vi "QuitTest.vi"(8 "error in":errorcluster caption="错误输入（无错误）", 11 "Com":refnum<visa-resource-name>) -> (0 "error out":errorcluster caption="错误输出", 3 "OK?":bool)   [LabVIEW 2013]
uses:
  Program Files/National Instruments/LabVIEW 2013/examples/Instrument IO/Serial/support/Serial - Settings.ctl
  <vilib>/Instr/_visa.llb/VISA Flush IO Buffer Mask.ctl
  <vilib>/Instr/_visa.llb/VISA Configure Serial Port (Instr).vi
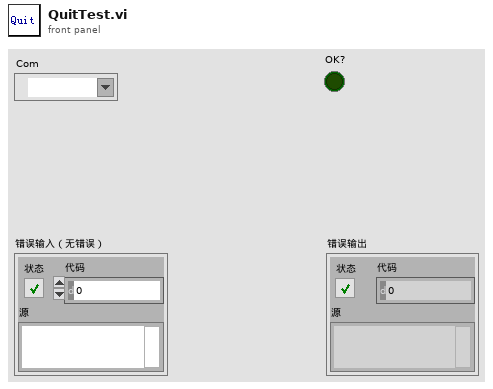
[diagram p1: front panel]
types:
  T1 = typedef "VISA Flush IO Buffer Mask.ctl" = u16
  T2 = typedef "Serial - Settings.ctl" = cluster{"波特率":u32, "数据比特":u16, "奇偶":enum16{"None", "Odd", "Even", "Mark", "Space"}, "停止位":u16, "流控制":u16}
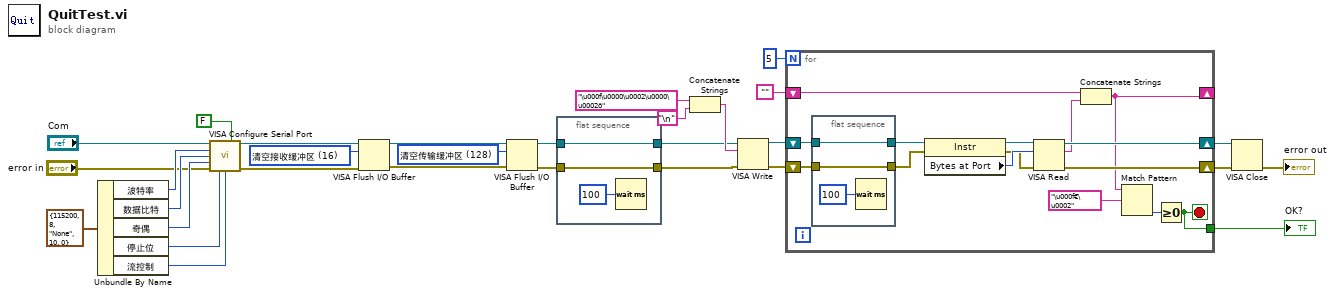
[diagram p0: block diagram]
diagram:
  w18 = T1 128 items=["清空接收缓冲区"=16, "向设备写入传输缓冲区"=32, "清空接收缓冲区（无I/O）"=64, "清空传输缓冲区"=128] ("Mask")
  w20 = T1 16 items=["清空接收缓冲区"=16, "向设备写入传输缓冲区"=32, "清空接收缓冲区（无I/O）"=64, "清空传输缓冲区"=128] ("Mask")
  n1 = Unbundle By Name(T2 {"波特率"=115200, "数据比特"=8, "奇偶"=enum."None", "停止位"=10, "流控制"=0} ("串口设置")) -> ("波特率"=w28:u32, "数据比特"=w27:u16, "奇偶"=w26:enum16{"None", "Odd", "Even", "Mark", "Space"}, "停止位"=w25:u16, "流控制"=w24:u16)
  n2 = call-poly "VISA Configure Serial Port"("VISA resource name"="Com", "Enable Termination\nChar (T)"=FALSE ("Enable Termination\nChar (T)"), "baud rate (9600)"=w28, "data bits (8)"=w27, "parity (0:none)"=w26, "error in (no error)"="error in", "stop bits (10: 1 bit)"=w25, "flow control (0:none)"=w24) -> ("VISA resource name out"=w22:refnum<visa-resource-name>, "error out"=w21:errorcluster)  [unwired: 6 in]
  n3 = VISA Flush I/O Buffer(VISA resource name=w22, mask (16)=w20, error in (no error)=w21) -> (VISA resource name out=w19:refnum<visa-resource-name>, error out=w17:errorcluster)
  n4 = VISA Flush I/O Buffer(VISA resource name=w19, mask (16)=w18, error in (no error)=w17) -> (VISA resource name out=w5:refnum<visa-resource-name>, error out=w2:errorcluster)
  n5 = flat-sequence {
    tunnel: w5 -> [w33]
    tunnel: [w33] -> w4
    tunnel: [w32] -> w3
    tunnel: w2 -> [w32]
    frame #0 {
      n6 = Wait (ms)(milliseconds to wait=u32 100 ("等待时间（毫秒）")) -> ()  [unwired: 1 out]
    }
  }
  n7 = Concatenate Strings("\u000f\u0000\u0002\u0000\u0002ð", "\n") -> (w16:string)
  n8 = VISA Write(VISA resource name=w4, write buffer=w16, error in (no error)=w3) -> (VISA resource name out=w14:refnum<visa-resource-name>, error out=w13:errorcluster)  [unwired: 1 out]
  n9 = for {
    N: 5 -> [_]
    shift-right: [w41] -> w12
    shift-left: w14 -> [w48]
    shift-right: [w40] -> w11
    shift-left: w13 -> [w47]
    shift-right: [w36] -> _
    shift-left: "" -> [w37]
    tunnel: [w34] -> w8
    stop <- w34 stop-if-true
    n10 = flat-sequence {
      tunnel: w48 -> [w51]
      tunnel: w47 -> [w50]
      tunnel: [w51] -> w46
      tunnel: [w50] -> w45
      frame #0 {
        n11 = Wait (ms)(milliseconds to wait=u32 100 ("等待时间（毫秒）")) -> ()  [unwired: 1 out]
      }
    }
    n12 = property class="Instr"(reference=w46, error in=w45) -> (reference out=w43:refnum<visa-resource-name>, error out=w42:errorcluster, "Bytes at Port"=w44:u32)
    n13 = VISA Read(VISA resource name=w43, byte count=w44, error in (no error)=w42) -> (VISA resource name out=w41:refnum<visa-resource-name>, read buffer=w38:string, error out=w40:errorcluster)  [unwired: 1 out]
    n14 = Concatenate Strings(w37, w38) -> (w36:string)
    n15 = Match Pattern(string=w36, regular expression="\u000f€\u0002") -> (offset past match=w35:i32)  [unwired: 1 in, 3 out]
    n16 = Greater Or Equal To 0?(x=w35) -> (x >= 0?=w34:bool)
  }
  "OK?" <- w8
  n17 = VISA Close(VISA resource name=w12, error in (no error)=w11) -> (error out=→"error out":errorcluster)
